vi "Triple Gaussian fitting model.vi"(3 "output control":T1 caption="输出控制", 4 "data":variant caption="数据", 5 "X":dbl[](array[numeric]), 6 "a":dbl[](array[numeric])) -> (0 "error out":errorcluster caption="错误输出", 1 "f'(X,a)":dbl[][](array[numeric]), 2 "f(X,a)":dbl[](array[numeric]))   [LabVIEW 2013]
doc: "This template is the starting point for creating a model function to be passed to the Nonlinear Curve Fit.vi."
uses:
  <vilib>/gmath/NumericalOptimization/LM_output select.ctl
  <vilib>/gmath/NI_Gmath.lvlib
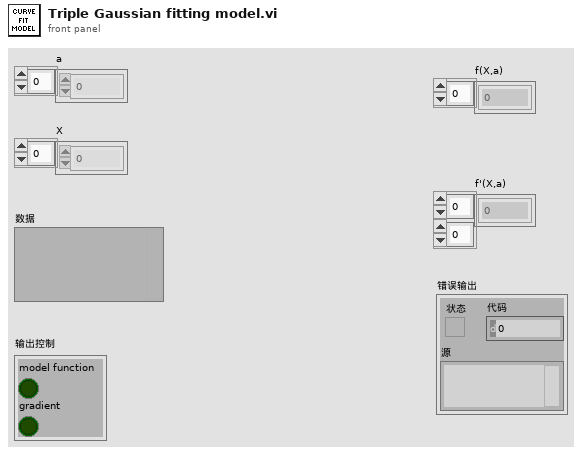
[diagram p1: front panel]
types:
  T1 = typedef "NI_Gmath.lvlib/LM_output select.ctl" = cluster{"model function":bool, "gradient":bool}
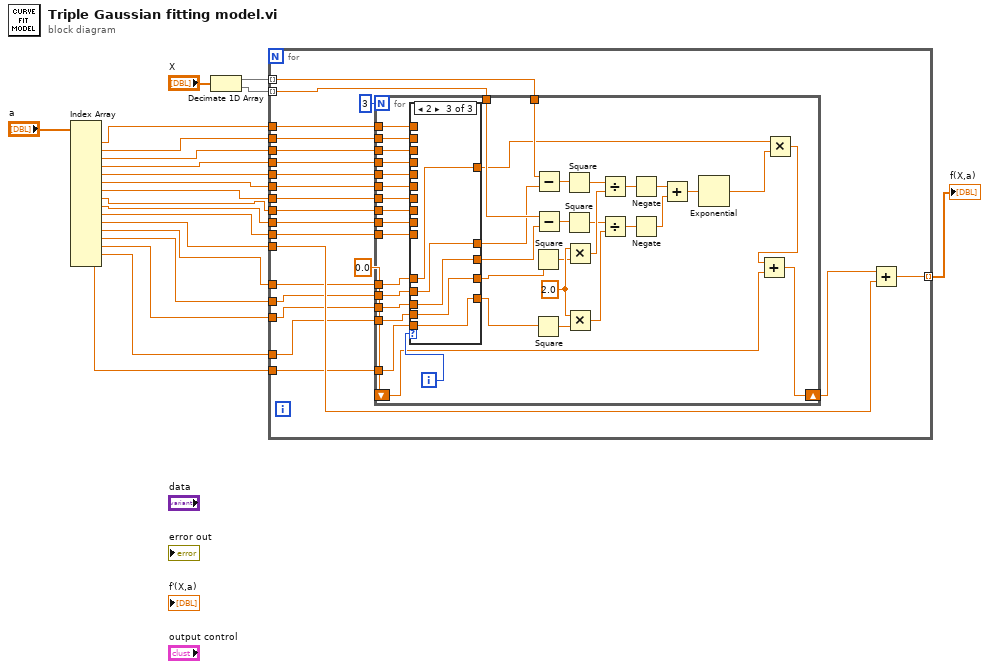
[diagram p0: block diagram]
diagram:
  n1 = Index Array(array="a") -> (element #1=w20:dbl, element #2=w19:dbl, element #3=w18:dbl, element #4=w17:dbl, element #5=w16:dbl, element #6=w14:dbl, element #7=w11:dbl, element #8=w10:dbl, element #9=w9:dbl, element #10=w8:dbl, element #11=w7:dbl, element #12=w3:dbl, element #13=w2:dbl, element #14=w1:dbl, element #15=w4:dbl, element #16=w5:dbl)  [unwired: 16 in]
  n2 = Decimate 1D Array("X") -> (w13:dbl[], w12:dbl[])
  n3 = for {
    tunnel: w20 -> [w42]
    tunnel: w19 -> [w41]
    tunnel: w18 -> [w40]
    tunnel: w17 -> [w39]
    tunnel: w16 -> [w38]
    tunnel: w12 -> [w31] mode=indexing
    tunnel: w14 -> [w37]
    tunnel: w13 -> [w32] mode=indexing
    tunnel: w11 -> [w36]
    tunnel: w10 -> [w35]
    tunnel: w9 -> [w34]
    tunnel: w8 -> [w33]
    tunnel: w7 -> [w29]
    tunnel: [w27] -> w6 mode=indexing
    tunnel: w5 -> [w22]
    tunnel: w4 -> [w23]
    tunnel: w3 -> [w26]
    tunnel: w2 -> [w25]
    tunnel: w1 -> [w24]
    n4 = for {
      N: 3 -> [_]
      tunnel: w42 -> [w69]
      tunnel: w41 -> [w68]
      tunnel: w40 -> [w67]
      tunnel: w39 -> [w66]
      tunnel: w38 -> [w65]
      tunnel: w37 -> [w64]
      tunnel: w36 -> [w63]
      tunnel: w35 -> [w62]
      tunnel: w34 -> [w61]
      tunnel: w33 -> [w60]
      tunnel: w32 -> [w59]
      tunnel: w31 -> [w58]
      shift-right: [w50] -> w28
      shift-left: 0.0 -> [w49]
      tunnel: w26 -> [w48]
      tunnel: w25 -> [w47]
      tunnel: w24 -> [w46]
      tunnel: w23 -> [w45]
      tunnel: w22 -> [w44]
      i -> [w70]
      w82 = 2.0 ("x")
      n5 = case shown="2" w70 {
        tunnel: w69 -> [w89 _ _]
        tunnel: w68 -> [w88 _ _]
        tunnel: w67 -> [w87 _ _]
        tunnel: w66 -> [w86 _ _]
        tunnel: w65 -> [w85 _ _]
        tunnel: w64 -> [_ w90 _]
        tunnel: w63 -> [_ w91 _]
        tunnel: w62 -> [_ w92 _]
        tunnel: w61 -> [_ w93 _]
        tunnel: w60 -> [_ w94 _]
        tunnel: [w88 w91 w98] -> w57
        tunnel: [w87 w92 w97] -> w56
        tunnel: [w86 w93 w96] -> w55
        tunnel: [w85 w94 w95] -> w54
        tunnel: [w89 w90 w99] -> w52
        tunnel: w48 -> [_ _ w99]
        tunnel: w47 -> [_ _ w98]
        tunnel: w46 -> [_ _ w97]
        tunnel: w45 -> [_ _ w96]
        tunnel: w44 -> [_ _ w95]
        frame 0, Default {
        }
        frame 1 {
        }
        frame 2 {
        }
      }
      n6 = Square(x=w55) -> (x^2=w81:dbl)
      n7 = Square(x=w54) -> (x^2=w80:dbl)
      n8 = Subtract(x=w59, y=w57) -> (x-y=w84:dbl)
      n9 = Subtract(x=w58, y=w56) -> (x-y=w83:dbl)
      n10 = Square(x=w84) -> (x^2=w79:dbl)
      n11 = Square(x=w83) -> (x^2=w77:dbl)
      n12 = Multiply(x=w82, y=w81) -> (x*y=w78:dbl)
      n13 = Multiply(x=w82, y=w80) -> (x*y=w76:dbl)
      n14 = Divide(x=w79, y=w78) -> (x/y=w75:dbl)
      n15 = Divide(x=w77, y=w76) -> (x/y=w74:dbl)
      n16 = Negate(x=w75) -> (-x=w73:dbl)
      n17 = Negate(x=w74) -> (-x=w72:dbl)
      n18 = Add(x=w73, y=w72) -> (x+y=w71:dbl)
      n19 = Exponential(1:w71) -> (0:w53:dbl)
      n20 = Multiply(x=w52, y=w53) -> (x*y=w51:dbl)
      n21 = Add(x=w51, y=w49) -> (x+y=w50:dbl)
    }
    n22 = Add(x=w28, y=w29) -> (x+y=w27:dbl)
  }
  "f(X,a)" <- w6
